vi "Test Set Port Status Comm.vi"(8 "error in (no error)":errorcluster, 11 "TestCase in":refnum<class "Test Set Port Status Command.lvclass">) -> (0 "error out":errorcluster, 3 "TestCase out":refnum<class "Test Set Port Status Command.lvclass">)   [LabVIEW 2020, in "Test Set Port Status Command.lvclass"]
uses:
  Test Set Port Status Command.lvclass
  Implementations/Simulado/Simulado.lvclass
  <vilib>/addons/_JKI Toolkits/VI Tester/TestCase.llb/TestCase.lvclass
  C:/Program Files (x86)/National Instruments/LabVIEW 2020/vi.lib/addons/_JKI Toolkits/VI Tester/TestCase.llb/TestCase.lvclass
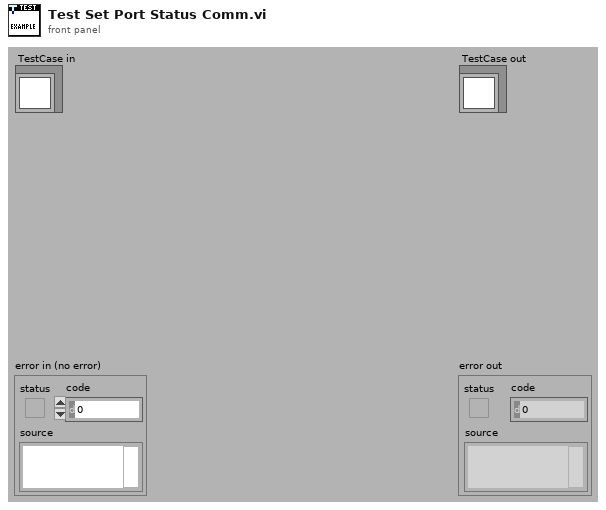
[diagram p1: front panel]
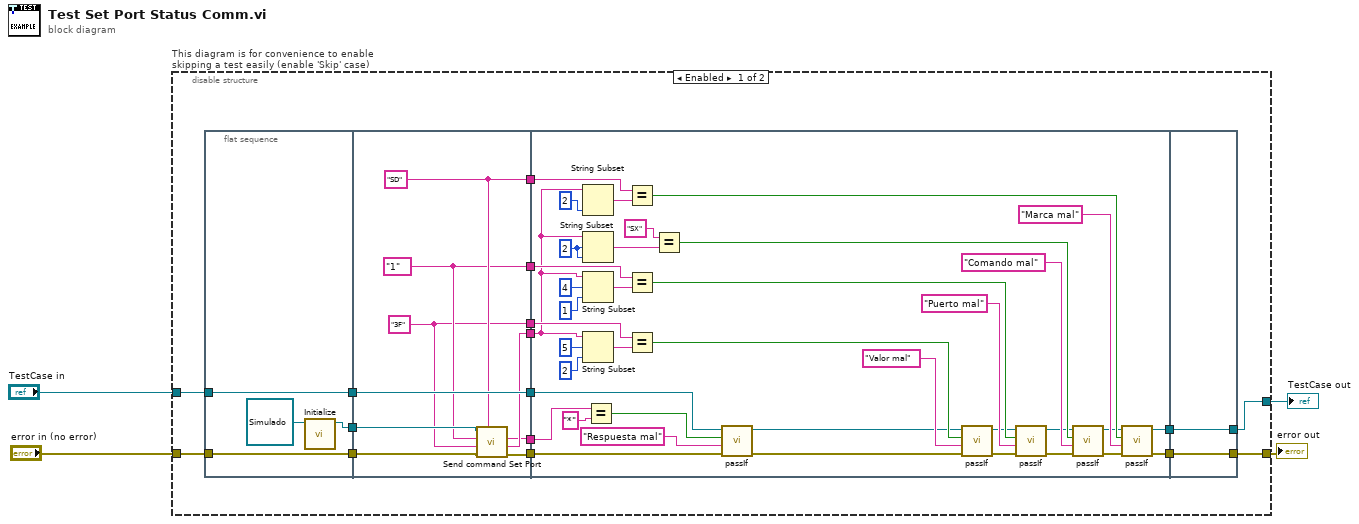
[diagram p0: block diagram]
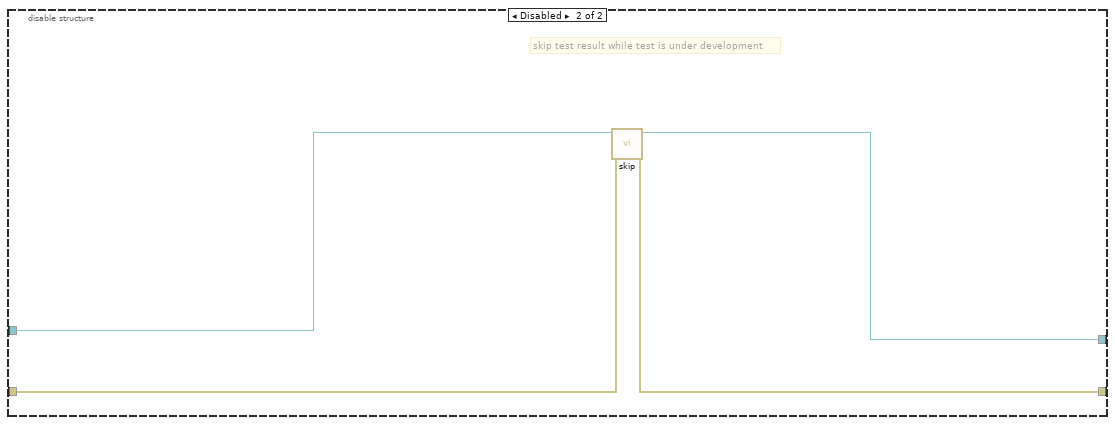
[diagram p2: hidden frame]
diagram:
  n1 = disable-structure "This diagram is for convenience to enable skipping a test easily (enable 'Skip' case)" shown="Enabled" {
    disable-tunnel: "TestCase in" -> [w6 w78]
    disable-tunnel: [w8 w76] -> w1
    disable-tunnel: [w7 w77] -> w3
    disable-tunnel: "error in (no error)" -> [w5 w75]
    frame Enabled {
      n2 = flat-sequence {
        tunnel: w6 -> [w24]
        tunnel: [w24] -> w20
        tunnel: w5 -> [w23]
        tunnel: [w23] -> w19
        tunnel: [w21] -> w18
        tunnel: [w33] -> w17
        tunnel: w20 -> [w33]
        tunnel: [w32] -> w16
        tunnel: w19 -> [w31]
        tunnel: w18 -> [w28]
        tunnel: [w30] -> w15
        tunnel: [w29] -> w14
        tunnel: [w27] -> w13
        tunnel: [w26] -> w12
        tunnel: [w25] -> w11
        tunnel: [w69] -> w10
        tunnel: w17 -> [w56]
        tunnel: [w68] -> w9
        tunnel: w16 -> [w55]
        tunnel: w15 -> [w36]
        tunnel: w14 -> [w58]
        tunnel: w13 -> [w70]
        tunnel: w12 -> [w47]
        tunnel: w11 -> [w41]
        tunnel: [w74] -> w8
        tunnel: w10 -> [w74]
        tunnel: [w73] -> w7
        tunnel: w9 -> [w73]
        frame #0 {
          n3 = call-dynamic "Initialize.vi"("object in"=refnum<class "Simulado.lvclass"> refnum ("Simulado.lvclass")) -> ("object out"=w21:refnum<class "Simulado.lvclass">)  [unwired: 9 in, 1 out]
        }
        frame #1 {
          w25 = "3F" ("Pin")
          w26 = "1" ("Puerto")
          w27 = "SD" ("Marca")
          n4 = call-dynamic "Send command Set Port.vi"("Marca"=w27, "error in (no error)"=w31, "Valor HEX"=w25, "Puerto"=w26, "Simulado in"=w28) -> ("error out"=w32:errorcluster, "Command"=w30:string, "Expected response"=w29:string)  [unwired: 3 in, 1 out]
        }
        frame #2 {
          w65 = 2 ("length (rest)")
          n5 = String Subset(string=w36, length (rest)=2 ("length (rest)")) -> (substring=w71:string)  [unwired: 1 in]
          n6 = String Subset(string=w36, offset (0)=w65, length (rest)=w65) -> (substring=w64:string)
          n7 = String Subset(string=w36, offset (0)=4, length (rest)=1 ("length (rest)")) -> (substring=w52:string)
          n8 = String Subset(string=w36, offset (0)=5, length (rest)=2 ("length (rest)")) -> (substring=w44:string)
          n9 = Equal?(x=w58, y="*") -> (x = y?=w54:bool)
          n10 = Equal?(x=w70, y=w71) -> (x = y?=w67:bool)
          n11 = Equal?(x=w47, y=w52) -> (x = y?=w46:bool)
          n12 = Equal?(x=w41, y=w44) -> (x = y?=w38:bool)
          n13 = Equal?(x="SX", y=w64) -> (x = y?=w60:bool)
          n14 = call-dynamic "passIf.vi"("error in (no error)"=w55, "message (\"\")"="Respuesta mal" ("message (\"\")"), "pass"=w54, "TestCase in"=w56) -> ("error out"=w34:errorcluster, "TestCase out"=w35:refnum<class "Test Set Port Status Command.lvclass">)  [unwired: 6 in]
          n15 = call-dynamic "passIf.vi"("error in (no error)"=w34, "message (\"\")"="Valor mal" ("message (\"\")"), "pass"=w38, "TestCase in"=w35) -> ("error out"=w40:errorcluster, "TestCase out"=w39:refnum<class "Test Set Port Status Command.lvclass">)  [unwired: 6 in]
          n16 = call-dynamic "passIf.vi"("error in (no error)"=w40, "message (\"\")"="Puerto mal" ("message (\"\")"), "pass"=w46, "TestCase in"=w39) -> ("error out"=w50:errorcluster, "TestCase out"=w49:refnum<class "Test Set Port Status Command.lvclass">)  [unwired: 6 in]
          n17 = call-dynamic "passIf.vi"("error in (no error)"=w50, "message (\"\")"="Comando mal" ("message (\"\")"), "pass"=w60, "TestCase in"=w49) -> ("error out"=w61:errorcluster, "TestCase out"=w62:refnum<class "Test Set Port Status Command.lvclass">)  [unwired: 6 in]
          n18 = call-dynamic "passIf.vi"("error in (no error)"=w61, "message (\"\")"="Marca mal" ("message (\"\")"), "pass"=w67, "TestCase in"=w62) -> ("error out"=w68:errorcluster, "TestCase out"=w69:refnum<class "Test Set Port Status Command.lvclass">)  [unwired: 6 in]
        }
        frame #3 {
        }
      }
    }
    frame Disabled {
      # "skip test result while test is under development"
      n19 = call <vilib>:"skip.vi"("error in (no error)"=w75, "TestCase in"=w78) -> ("error out"=w77:errorcluster, "TestCase out"=w76:refnum<class "Test Set Port Status Command.lvclass">)  [unwired: 8 in]
    }
  }
  "error out" <- w3
  "TestCase out" <- w1
